vi "公式读取.vi"(8 "error in (no error)":errorcluster caption="错误输入（无错误）", 9 "量程":enum16{"低量程", "高量程"}(ring), 10 "测量模式":T1(ring), 11 "测量参数":enum16{"CODMn"}(ring)) -> (0 "error out":errorcluster caption="错误输出", 3 "公式":cluster{"X^2":dbl, "X":dbl, "b":dbl})   [LabVIEW 2016, in "斯坦道CODMn新电路板.lvlib"]
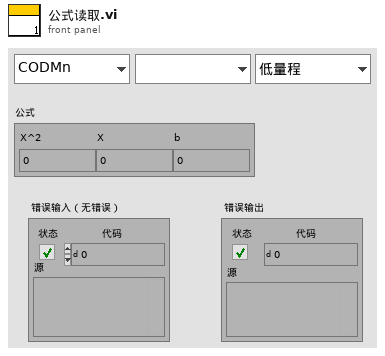
[diagram p1: front panel]
types:
  T1 = enum16{"", "水样测量", "标样核查", "零点核查", "跨度核查", "空白测试", "平行样测试", "加标回收"}
  T2 = cluster{"FLOAT[0]":sgl, "FLOAT[1]":sgl, "FLOAT[2]":sgl}
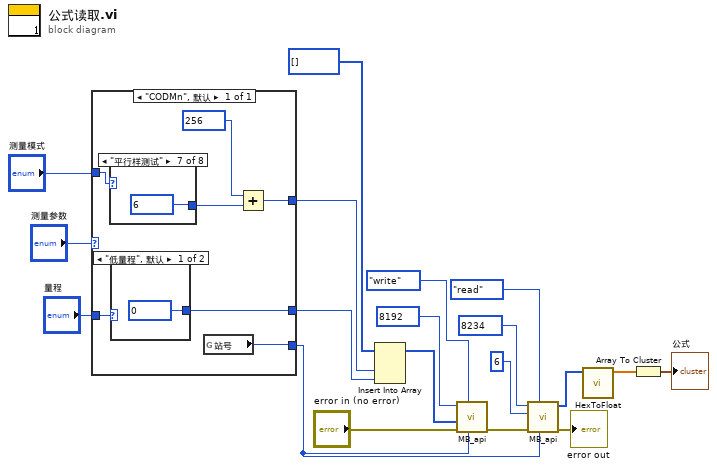
[diagram p0: block diagram]
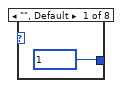
[diagram p2: hidden frame]
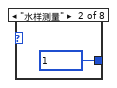
[diagram p3: hidden frame]
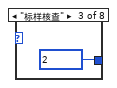
[diagram p4: hidden frame]
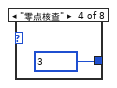
[diagram p5: hidden frame]
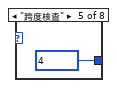
[diagram p6: hidden frame]
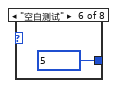
[diagram p7: hidden frame]
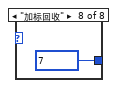
[diagram p8: hidden frame]
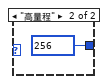
[diagram p9: hidden frame]
diagram:
  n1 = case shown="\"CODMn\", 默认" "测量参数" {
    tunnel: "测量模式" -> [w20]
    tunnel: "量程" -> [w26]
    tunnel: [w22] -> w6
    tunnel: [w23] -> w10
    tunnel: [w25] -> w9
    frame "CODMn", Default {
      n2 = case shown="\"平行样测试\"" w20 {
        tunnel: [u16 1 ("starting address") u16 1 ("starting address") u16 2 ("starting address") u16 3 ("starting address") u16 4 ("starting address") u16 5 ("starting address") u16 6 ("starting address") u16 7 ("starting address")] -> w21
        frame "", Default {
        }
        frame "水样测量" {
        }
        frame "标样核查" {
        }
        frame "零点核查" {
        }
        frame "跨度核查" {
        }
        frame "空白测试" {
        }
        frame "平行样测试" {
        }
        frame "加标回收" {
        }
      }
      n3 = case shown="\"低量程\", 默认" w26 {
        tunnel: [u16 0 ("starting address") u16 256 ("starting address")] -> w25
        frame "低量程", Default {
        }
        frame "高量程" {
        }
      }
      n4 = global read "CODMn断电保存全局变量.vi" "站号"() -> (w22:u16)
      n5 = Add(x=u16 256 ("starting address"), y=w21) -> (x+y=w23:u16)
    }
  }
  n6 = Insert Into Array(array=u16[] [] ("数组"), new element #1=w10, new element #2=w9) -> (w2:u16[])  [unwired: 1 in]
  n7 = call "MB_api.vi"("Slave ID"=w6, "STEP"=enum16{"open", "read", "write", "close"}."write", "Error in"="error in (no error)", "values"=w2, "starting address"=u16 8192) -> ("error out"=w5:errorcluster)  [unwired: 4 in, 2 out]
  n8 = call "MB_api.vi"("Slave ID"=w6, "STEP"=enum16{"open", "read", "write", "close"}."read", "Error in"=w5, "quantity"=u16 6, "starting address"=u16 8234) -> ("error out"=→"error out":errorcluster, "Registers"=w16:u16[])  [unwired: 4 in, 1 out]
  n9 = call "HexToFloat.vi"("数组"=w16) -> ("FLOAT"=w15:sgl[])  [unwired: 10 in]
  n10 = Array To Cluster(array=w15) -> (cluster=→"公式":T2)
